vi "SVN Version.vi"(8 "error in (no error)":errorcluster) -> (0 "error out":errorcluster, 1 "Successful version check":bool, 2 "Revision":i32, 3 "standard output":string)   [LabVIEW 2012, in "Design Server.lvlib"]
uses:
  Design Server.lvlib
  Folders.ctl
  ReadWrite.ctl
panel:
  in  "Update SVN (600s)":dbl=600.0
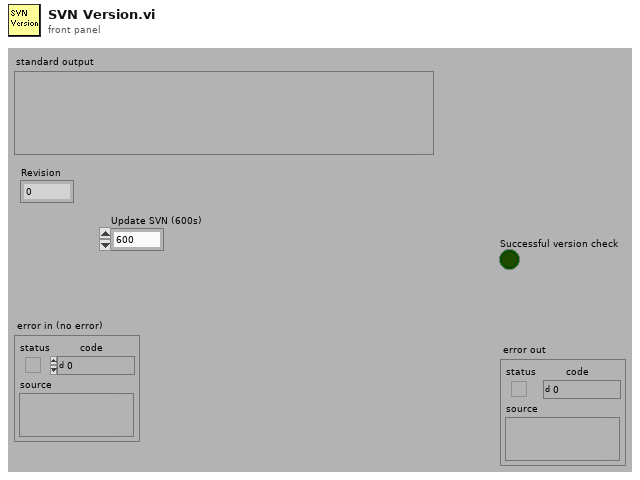
[diagram p1: front panel]
types:
  T1 = typedef "ReadWrite.ctl" = enum16{"Read", "Write"}
  T2 = typedef "Design Server.lvlib/Folders.ctl" = enum16{"MathcadMethods", "RequestedDesigns", "CompletedDesigns", "MathcadCode", "CollabnetSVN.exe"}
  T3 = typedef "SVN.ctl" = cluster{"Mathcad Code Repository":string, "Username":string, "Password":string, "Method file names (w extension)":string}
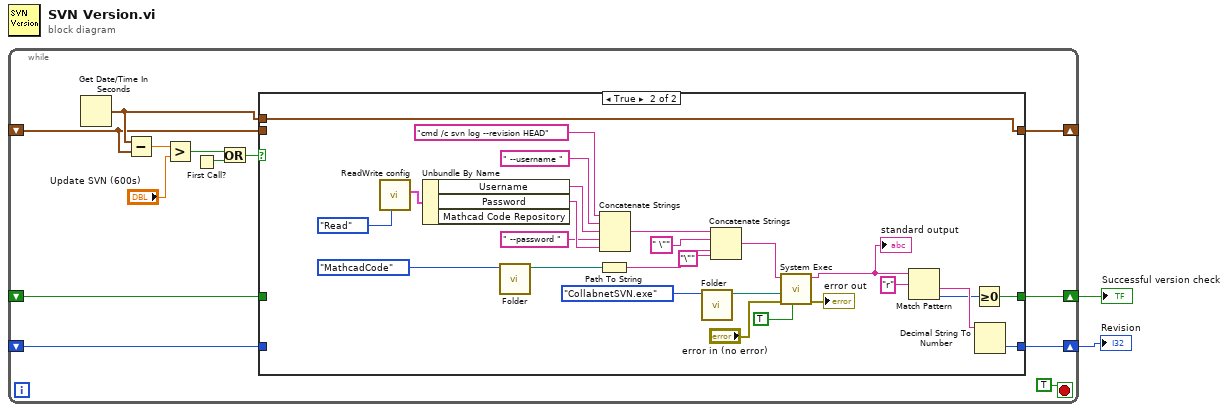
[diagram p0: block diagram]
diagram:
  n1 = while {
    shift-right: [w15] -> w1
    shift-left: _ -> [w6]
    shift-right: [w14] -> w2
    shift-left: _ -> [w7]
    shift-right: [w13] -> _
    shift-left: _ -> [w8]
    stop <- TRUE stop-if-true
    n2 = Get Date/Time In Seconds() -> (seconds since 1Jan1904=w9:timestamp)
    n3 = Subtract(x=w9, y=w8) -> (x-y=w12:dbl)
    n4 = Greater?(x=w12, y="Update SVN (600s)") -> (0:w10:bool)
    n5 = First Call?() -> (First Call?: T/F=w3:bool)
    n6 = Or(x=w10, y=w3) -> (x .or. y?=w4:bool)
    n7 = case shown="True" w4 {
      tunnel: [w16 w21] -> w15
      tunnel: [w17 w20] -> w14
      tunnel: [w18 w19] -> w13
      tunnel: w9 -> [_ w19]
      tunnel: w8 -> [w18 _]
      tunnel: w7 -> [w17 _]
      tunnel: w6 -> [w16 _]
      frame False {
      }
      frame True {
        n8 = call "ReadWrite config.vi"("Config"=ReadWrite."Read") -> ("SVN"=w30:T3)  [unwired: 7 in, 3 out]
        n9 = Unbundle By Name(w30) -> ("Username"=w27:string, "Password"=w29:string)  [unwired: 1 out]
        n10 = call "Folder.vi"("Folders"=Folders."MathcadCode") -> ("FolderPath"=w33:path)  [unwired: 8 in, 2 out]
        n11 = Path To String(path=w33) -> (string=w43:string)
        n12 = Concatenate Strings("cmd /c svn log --revision HEAD" ("command"), " --username " ("string"), w27, " --password " ("string"), w29) -> (w23:string)
        n13 = call "Folder.vi"("Folders"=Folders."CollabnetSVN.exe") -> ("FolderPath"=w31:path)  [unwired: 8 in, 2 out]
        n14 = Concatenate Strings(w23, " \"" ("string"), w43, "\"" ("string")) -> (w36:string)
        n15 = call <vilib>:"System Exec.vi"("run minimized? (F)"=TRUE, "error in (no error)"="error in (no error)", "working directory"=w31, "command line"=w36) -> ("error out"=→"error out":errorcluster, "standard output"=w40:string)  [unwired: 4 in, 2 out]
        "standard output" <- w40
        n16 = Match Pattern(string=w40, regular expression="r") -> (after substring=w38:string, offset past match=w22:i32)  [unwired: 1 in, 2 out]
        n17 = Greater Or Equal To 0?(x=w22) -> (x >= 0?=w20:bool)
        n18 = Decimal String To Number(string=w38) -> (number=w21:i32)  [unwired: 2 in, 1 out]
      }
    }
  }
  "Revision" <- w1
  "Successful version check" <- w2
